vi "Actor Core.vi"(8 "error in":errorcluster, 11 "Calculadora in":refnum<class "Calculadora.lvclass">) -> (0 "error out":errorcluster, 3 "Actor out":refnum<class "Actor.lvclass">)   [LabVIEW 2020, in "Calculadora.lvlib" / "Calculadora.lvclass"]
doc: "(<B>Filename</B>: Actor Framework.lvlib:Actor.lvclass:Actor Core.vi)\n\nReceives messages to the actor, reacts to them, and initiates any error handling that may shut the actor down.\n\nDescendant classes may override this VI to append parallel tasks for the actor to complete while it handles messages. Overrides use the Call Parent Class Method node."
uses:
  Calculadora.lvclass
  C:/Program Files (x86)/National Instruments/LabVIEW 2020/vi.lib/ActorFramework/Actor/Actor.lvclass
  <vilib>/ActorFramework/Actor/Actor.lvclass
  <vilib>/ActorFramework/Actor/Actor.lvclass/Actor.ctl
  <vilib>/ActorFramework/Message Enqueuer/Message Enqueuer.lvclass/Message Enqueuer.ctl
  Calculadora.lvclass/Calculadora.ctl
  Calculadora Messages/Set Numero A Msg/Set Numero A Msg.lvclass/Set Numero A Msg.ctl
  Calculadora Messages/Set Numero B Msg/Set Numero B Msg.lvclass/Set Numero B Msg.ctl
  <vilib>/ActorFramework/Message Enqueuer/Init from Existing Queue.vi
  <vilib>/ActorFramework/Message Enqueuer/Enqueue.vi
  Calculadora Messages/Set Numero A Msg/Set Numero A Msg.lvclass
  C:/Program Files (x86)/National Instruments/LabVIEW 2020/vi.lib/ActorFramework/Message/Message.lvclass
  Calculadora Messages/Set Numero B Msg/Set Numero B Msg.lvclass
  <vilib>/ActorFramework/Stop Msg/Stop Msg.lvclass
  Calculadora Messages/Suma Msg/Suma Msg.lvclass
  Calculadora Messages/Resta Msg/Resta Msg.lvclass
  Calculadora Messages/Multiplicacion Msg/Multiplicacion Msg.lvclass
  Calculadora Messages/Division Msg/Division Msg.lvclass
  <vilib>/ActorFramework/Message Priority Queue/Priority Enqueue.vi
  <vilib>/ActorFramework/Message Enqueuer/Message Enqueuer.lvclass
panel:
  out "Resultado":dbl
  in  "Division":bool
  in  "Multiplicacion":bool
  in  "Resta":bool
  in  "Suma":bool
  in  "Stop":bool
  in  "B":dbl(slide) scale=0.0..10.0
  in  "A":dbl(slide) scale=0.0..10.0
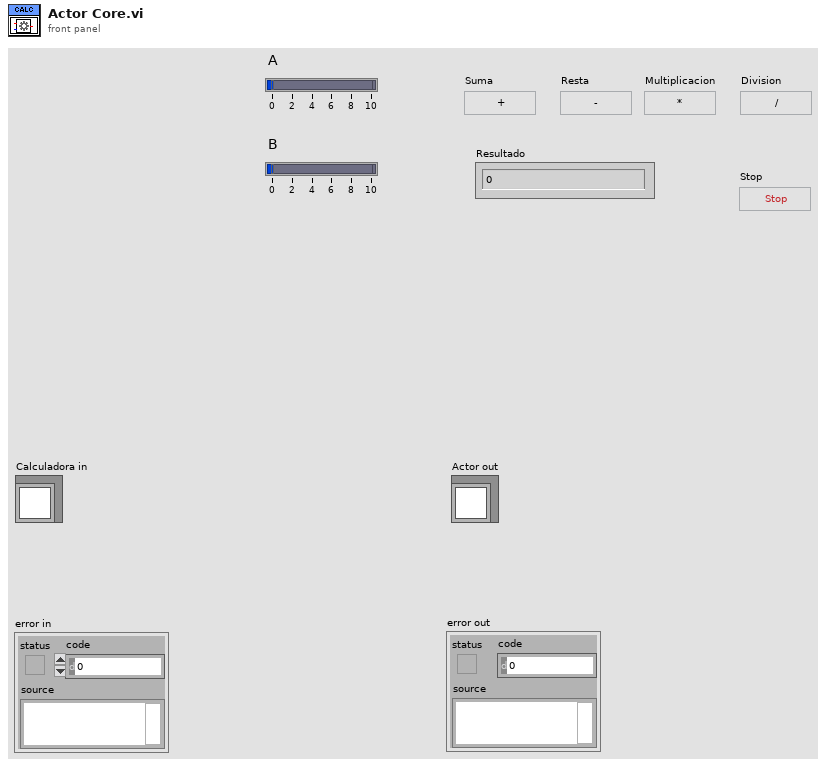
[diagram p1: front panel]
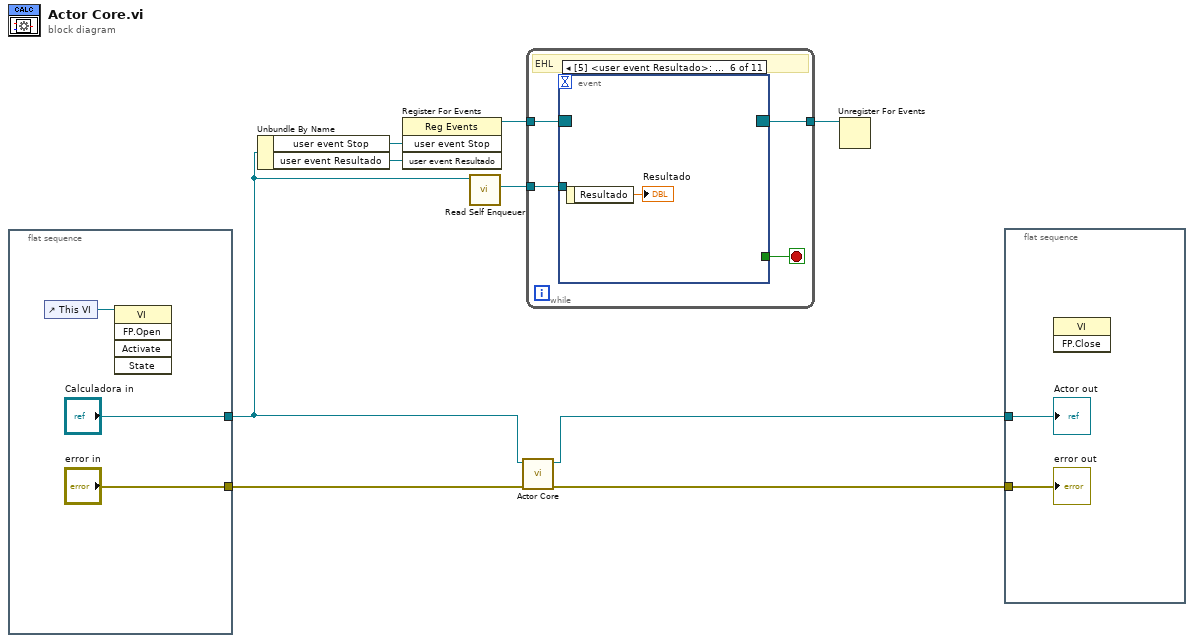
[diagram p0: block diagram]
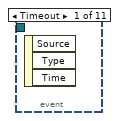
[diagram p2: hidden frame]
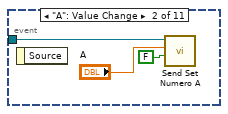
[diagram p3: hidden frame]
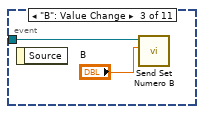
[diagram p4: hidden frame]
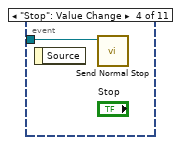
[diagram p5: hidden frame]
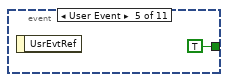
[diagram p6: hidden frame]
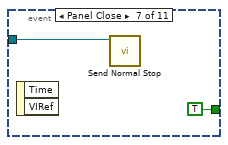
[diagram p7: hidden frame]
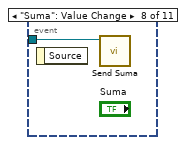
[diagram p8: hidden frame]
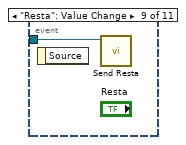
[diagram p9: hidden frame]
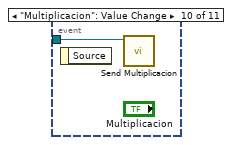
[diagram p10: hidden frame]
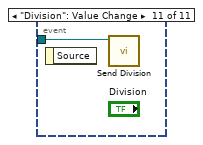
[diagram p11: hidden frame]
diagram:
  n1 = flat-sequence {
    tunnel: ["error in"] -> w7
    tunnel: ["Calculadora in"] -> w2
    frame #0 {
      n2 = control-ref of="This VI"() -> (w10:refnum<vi>)
      n3 = invoke class="VI" method="FP.Open"(reference=w10) -> ()  [unwired: 4 in, 5 out]
    }
  }
  n4 = Unbundle By Name(w2) -> ("user event Stop"=w4:refnum<user-event>, "user event Resultado"=w1:refnum<user-event>)
  n5 = register-events(w4, w1) -> (reference out=w5:refnum<event-registration>)  [unwired: 2 in, 1 out]
  n6 = call <vilib>:"Read Self Enqueuer.vi"("Actor"=w2) -> ("Self Enqueuer"=w6:refnum<class "Message Enqueuer.lvclass">)  [unwired: 10 in]
  n7 = call-parent "Actor Core.vi"("error in"=w7, "Actor in"=w2) -> ("error out"=w9:errorcluster, "Actor out"=w8:refnum<class "Actor.lvclass">)  [unwired: 8 in]
  n8 = while {
    tunnel: w6 -> [w16]
    tunnel: w5 -> [w14]
    tunnel: [w13] -> w3
    stop <- w15 stop-if-true
    # "EHL"
    n9 = event shown="[5] <user event Resultado>: User Event" {
      selector: w14 -> [_ _ _ _ _ _ _ _ _ _ _]
      dyn-events: [_ _ _ _ _ _ _ _ _ _ _] -> w13
      timeout: _ -> [_ _ _ _ _ _ _ _ _ _ _]
      tunnel: w16 -> [_ w19 w20 w22 _ _ w26 w27 w28 w29 w30]
      tunnel: [_ _ _ _ TRUE ("Stop") _ TRUE ("Stop") _ _ _ _] -> w15
      event Timeout {
        n10 = event-data() -> ()  [unwired: 1 in, 3 out]
      }
      event "A": Value Change {
        n11 = event-data() -> ()  [unwired: 1 in, 1 out]
        n12 = call "Send Set Numero A.vi"("Boolean"=FALSE, "Numero A"="A", "Message Enqueuer"=w19) -> ()  [unwired: 7 in, 2 out]
      }
      event "B": Value Change {
        n13 = event-data() -> ()  [unwired: 1 in, 1 out]
        n14 = call "Send Set Numero B.vi"("Numero B"="B", "Message Enqueuer"=w20) -> ()  [unwired: 8 in, 2 out]
      }
      event "Stop": Value Change {
        n15 = event-data() -> ()  [unwired: 1 in, 1 out]
        n16 = call <vilib>:"Send Normal Stop.vi"("Message Enqueuer"=w22) -> ()  [unwired: 10 in, 1 out]
      }
      event User Event {
        n17 = event-data() -> ()  [unwired: 1 in, 1 out]
      }
      event User Event {
        n18 = event-data() -> ("Resultado"=→"Resultado":dbl)  [unwired: 1 in]
      }
      event Panel Close {
        n19 = event-data() -> ()  [unwired: 1 in, 2 out]
        n20 = call <vilib>:"Send Normal Stop.vi"("Message Enqueuer"=w26) -> ()  [unwired: 10 in, 1 out]
      }
      event "Suma": Value Change {
        n21 = event-data() -> ()  [unwired: 1 in, 1 out]
        n22 = call "Send Suma.vi"("Message Enqueuer"=w27) -> ()  [unwired: 9 in, 2 out]
      }
      event "Resta": Value Change {
        n23 = event-data() -> ()  [unwired: 1 in, 1 out]
        n24 = call "Send Resta.vi"("Message Enqueuer"=w28) -> ()  [unwired: 9 in, 2 out]
      }
      event "Multiplicacion": Value Change {
        n25 = event-data() -> ()  [unwired: 1 in, 1 out]
        n26 = call "Send Multiplicacion.vi"("Message Enqueuer"=w29) -> ()  [unwired: 9 in, 2 out]
      }
      event "Division": Value Change {
        n27 = event-data() -> ()  [unwired: 1 in, 1 out]
        n28 = call "Send Division.vi"("Message Enqueuer"=w30) -> ()  [unwired: 9 in, 2 out]
      }
    }
  }
  n29 = Unregister For Events(event registration refnum=w3) -> ()  [unwired: 1 in, 1 out]
  n30 = flat-sequence {
    tunnel: w9 -> [w32]
    tunnel: w8 -> [w31]
    frame #0 {
      n31 = invoke class="VI" method="FP.Close"() -> ()  [unwired: 3 in, 3 out]
      "error out" <- w32
      "Actor out" <- w31
    }
  }
